vi "NI9234_SUB-VI_INIT.vi"(4 "Sample Rate":dbl=1000.0, 8 "error in":errorcluster, 9 "IEPE Current value (A)":dbl=0.004 format="%#_13g", 10 "Sensitivity (mV/g)":dbl=50.0, 11 "Physical Channel":tag="Dev1/ai0") -> (0 "error out":errorcluster, 2 "Actual Sample Rate":dbl=1000.0000111176631 format="%0.2f", 3 "task out":refnum<k21>, 5 "min Acc Read":dbl, 7 "Max Acc Read":dbl)   [LabVIEW 2020]
uses:
  <vilib>/DAQmx/create/channels.llb/DAQmx Create Channel (AI-Acceleration-Accelerometer).vi
  <vilib>/DAQmx/configure/timing.llb/DAQmx Timing (Sample Clock).vi
  <resource>/objmgr/daqmx.rc
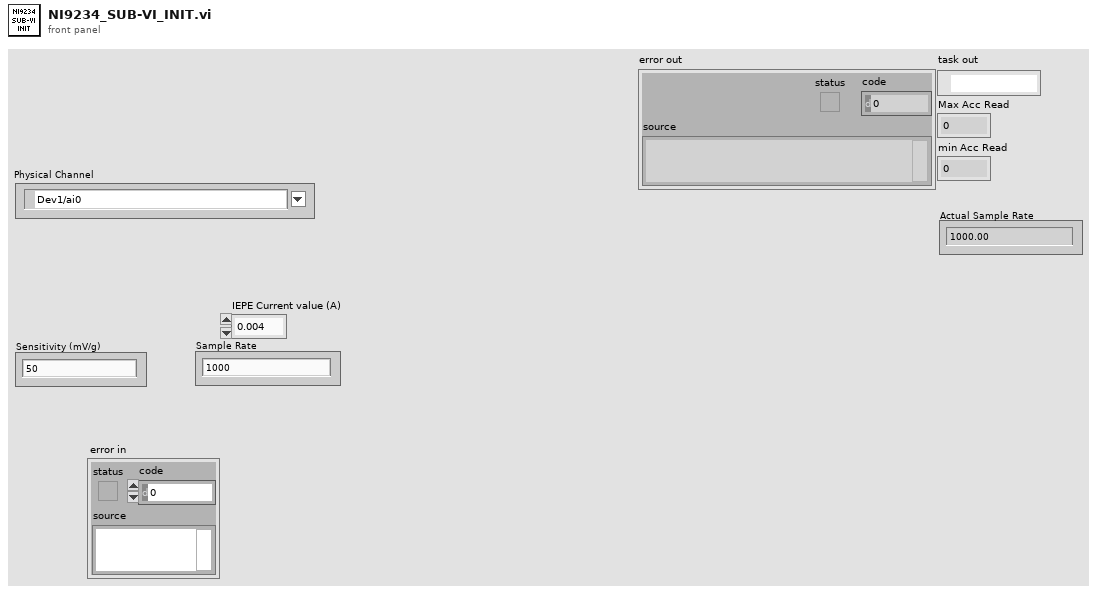
[diagram p1: front panel]
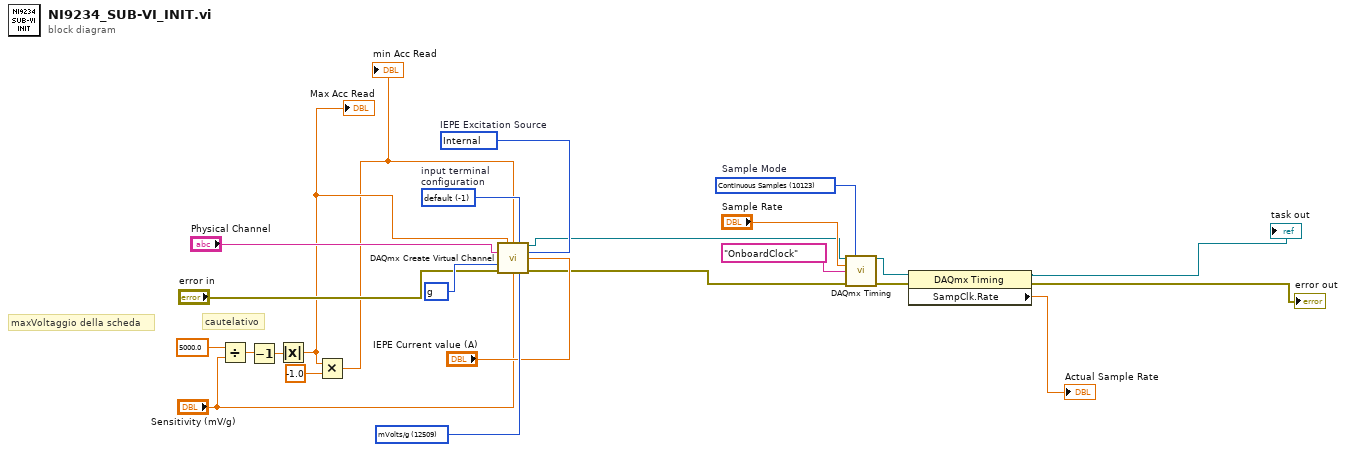
[diagram p0: block diagram]
diagram:
  w20 = 10200 items=["Internal"=10200, "External"=10167, "None"=10230]  # IEPE Excitation Source
  w19 = 10123 items=["Finite Samples"=10178, "Continuous Samples"=10123, "Hardware Timed Single Point"=12522]  # Sample Mode
  w24 = 12509 items=["mVolts/g"=12509, "Volts/g"=12510] ("Sensitivity Units")
  w23 = 10186 items=["g"=10186, "m/s^2"=12470, "in/s^2"=12471, "From Custom Scale"=10065] ("Acceleration Units")
  w22 = -1 items=["default"=-1, "RSE"=10083, "NRSE"=10078, "Differential"=10106, "Pseudodifferential"=12529]  # input terminal configuration
  # "cautelativo"
  # "maxVoltaggio della scheda"
  n1 = Divide(x=5000.0, y="Sensitivity (mV/g)") -> (x/y=w7:dbl)
  n2 = Decrement(x=w7) -> (x-1=w6:dbl)
  n3 = Absolute Value(x=w6) -> (abs(x)=w4:dbl)
  "Max Acc Read" <- w4
  n4 = Multiply(x=w4, y=-1.0) -> (x*y=w3:dbl)
  "min Acc Read" <- w3
  n5 = call-poly <vilib>:"DAQmx Create Virtual Channel.vi"("maximum value"=w4, "minimum value"=w3, "input terminal configuration"=w22, "physical channels"="Physical Channel", "current excitation source"=w20, "current excitation value"="IEPE Current value (A)", "units"=w23, "error in"="error in", "sensitivity"="Sensitivity (mV/g)", "sensitivity units"=w24) -> ("task out"=w11:refnum<k21>, "error out"=w16:errorcluster)  [unwired: 4 in]
  n6 = call-poly <vilib>:"DAQmx Timing.vi"("task/channels in"=w11, "sample mode"=w19, "rate"="Sample Rate", "source"=tag "OnboardClock" ("Sample Clock Source"), "error in"=w16) -> ("task out"=w14:refnum<k21>, "error out"=w10:errorcluster)  [unwired: 9 in]
  n7 = property class="DAQmx Timing"(reference=w14, error in=w10) -> (reference out=→"task out":refnum<k21>, error out=→"error out":errorcluster, "SampClk.Rate"=→"Actual Sample Rate":dbl)
